vi "Caraya Batch Testing.vi"(4 "Verbose":bool=TRUE, 5 "Silent":bool, 6 "Interactive":bool=TRUE, 7 "Inspect Recursively":bool=TRUE, 9 "Report name":string, 10 "Output Folder":path, 11 "Source Folder":path) -> (0 "error out":errorcluster, 3 "Test Runner":refnum<class "Test Runner.lvclass">)   [LabVIEW 2013]
uses:
  classes/Test Runner/Test Runner.lvclass
  Caraya.lvlib
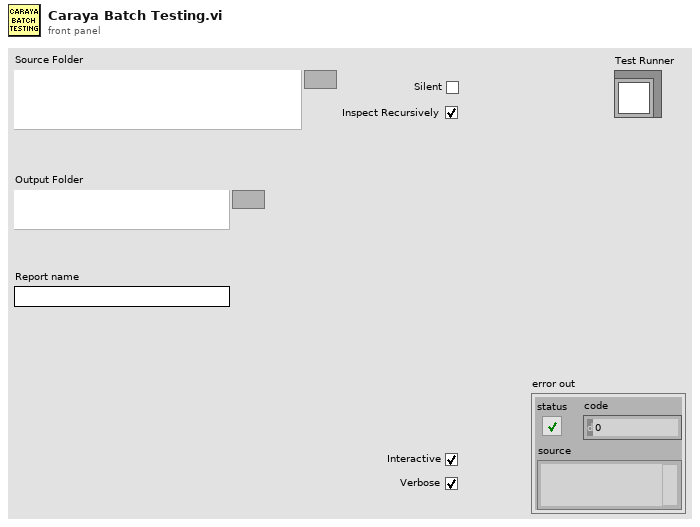
[diagram p1: front panel]
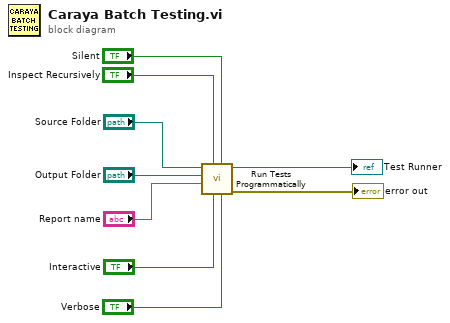
[diagram p0: block diagram]
diagram:
  n1 = call "Run Tests Programmatically.vi"("Verbose"="Verbose", "Silent"="Silent", "Interactive"="Interactive", "Inspect Recursively"="Inspect Recursively", "Report name"="Report name", "Output Folder"="Output Folder", "Source Folder"="Source Folder") -> ("error out"=→"error out":errorcluster, "Test Runner"=→"Test Runner":refnum<class "Test Runner.lvclass">)  [unwired: 3 in]
